vi "BonOMM-SAOMM.vi"() -> ()   [LabVIEW 2019]
uses:
  <vilib>/Utility/miscctls.llb/LVPointTypeDef.ctl
  <vilib>/Utility/miscctls.llb/LVRectTypeDef.ctl
  <vilib>/Analysis/baseanly.llb/Mean (DBL).vi
  SubVIs/Globals.vi
  <vilib>/Utility/config.llb/Read Key (Double).vi
  <vilib>/Utility/config.llb/Read Key (U32).vi
  <vilib>/Utility/config.llb/Read Key (I32).vi
  <vilib>/Utility/config.llb/Read Key (String).vi
  <vilib>/Utility/config.llb/Read Key (Boolean).vi
  SubVIs/Polymorphics/Num2littleEndian(DBL).vi
  SubVIs/Polymorphics/Num2littleEndian(U32).vi
  <vilib>/Instr/_visa.llb/VISA Configure Serial Port (Instr).vi
  SubVIs/Polymorphics/Num2littleEndian(U16).vi
  SubVIs/gfitsio/gfitsio-read-image-subset-sgl-2d.vi
  SubVIs/SAOMM/EXTRACT-DATA-UINT32.vi
  SubVIs/SAOMM/EXTRACT-DATA-UINT16.vi
  SubVIs/SAOMM/EXTRACT-DATA-DBL.vi
  <vilib>/Utility/config.llb/Write Key (Double).vi
  <vilib>/Utility/config.llb/NI_LVConfig.lvlib
  SubVIs/gfitsio/gfitsio.lvlib
  <vilib>/Analysis/NI_AALBase.lvlib
panel:
  in  "VarTab":T1(tab)
  in  "ProcessImage":bool
  out "MaskObjet":u8[][](graph)
  in  "SaveFalconProc":bool
  out "FalconProcData":u8[](array[numeric])
  in  "HexRAZ":bool
  out "Nb_FalconProc_demandé":u32
  in  "GetCommand":string
  out "XROIRef":dbl
  out "YROIRef":dbl
  out "XRefMin":dbl
  out "YRefMin":dbl
  out "XRefMax":dbl
  out "YRefMax":dbl
  out "ROIWidthMin":u16
  out "ROIHeightMin":u16
  out "ROIWidthMax":u16
  out "ROIHeightMax":u16
  out "Nb_Error (PrAMS)":i32
  out "Nb_Error (hex)":i32
  in  "QueryServoLevel":bool
  out "ROISizes":u16[](array[numeric])
  in  "ROIsurface":i32(ring) items=["2.6\" x 2.6\"", "5.2\" x 5.2\"", "7.7\" x 7.7\"", "10.3\" x 10.3\"", "12.9\" x 12.9\"", "20.6\" x 20.6\""]
  out "ROIXMin":u16
  out "ROIYMin":u16
  out "ROIXMax":u16
  out "ROIYMax":u16
  out "PixScale2":dbl=0.323 format="%.4f"
  out "Naxis2":u16=99
  out "Naxis1":u16=142
  out "PixScale1":dbl=0.323 format="%.4f"
  out "Déc étoile guide":dbl=89448.04336960503 caption="DEC" format="%<%H:%M:%S%0u>t"
  out "A.D. étoile guide":dbl=54197.70933641569 caption="RA" format="%<%H:%M:%S%0u>t"
  out "TmpFalcon":u32
  in  "Binning":u16(ring) items=["1 x 1"=1, "2 x 2"=2, "4 x 4"=4, "5 x 5"=5]
  out "FPGA Value":u16(ring) items=["Disabled", "Enabled", "Enabled & Deep Cooling", "Disabled (fan disabled)", "Enabled (fan disabled)", "Enabled & Deep Cooling (fan disabled)"]
  out "InstantFPS":dbl format="%.2f"
  out "HexapodQuery":u32
  out "EMGain":u16
  out "GetOptimalTime":u32
  in  "ImageFPS":dbl=1.0 min=1.0 max=30.0 step=1.0
  out "SetROITime":u32
  out "StartTime":u32
  out "StopTime":u32
  out "SetExpTime":u32
  out "ListenerExec":u32
  out "SetBinningTime":u32
  out "SetFPSTime":u32
  out "ImageWidth":u16
  out "ImageHeight":u16
  out "ROIXOffset":u16
  out "ROIYOffset":u16
  in  "ROIWidth":u16
  in  "ROIHeight":u16
  out "Nb_ACK (PrAMS)":i32
  out "ImageProcessing":u32
  out "FalconQuery":u32
  out "nDumped":i32
  in  "HexapodRefresh":bool
  in  "UpdateROI":bool
  in  "ClearDump":bool
  in  "FalconRefresh":bool
  out "Connexion":bool
  out "Lecture":bool
  out "Écriture":bool
  in  "FalconProcessed":bool
  out "Nb_ACK (hex)":i32
  in  "GetOptimal":bool
  in  "refresh":bool
  out "Nb_FalconProc_reçu":u32
  in  "SendHexOffset":bool caption="SEND Offset"
  out "ImageStat":T2 {"SNR" format="%0.2f"; "mean" format="%0.2f"; "Flux" format="%0.2f"; "Variance" format="%0.2f"; "median" format="%0.2f"}
  out "ImageBuffer":u16[][](graph)
  out "GE_Hex_V":dbl
  out "GE_Hex_U":dbl
  out "GE_Hex_Z":dbl
  out "GE_Hex_Y":dbl
  out "GE_Hex_X":dbl
  out "GE_TCS":bool
  in  "Mode Guidage et Dither":bool=TRUE
  out "MirFOV":dbl=54.5268 caption="Miroir FOV" format="%.2f"
  out "MirVig":dbl=54.5268 caption="Miroir + Vignetting" format="%.2f"
  out "Miroir":dbl=54.5268 format="%.2f"
  in  "ClickJOG":dbl=302.0 min=250.0 max=20000.0
  out "ActiveStages":string[](array[string])
  out "Focusing":bool=TRUE
  out "CurvCorrect":bool=TRUE
  out "CorrectXY":bool=TRUE
  out "CorrectZ":bool=TRUE
  out "MovingZ":bool=TRUE
  out "vitesse jog":dbl=302.0 caption="Vitesse jog" min=250.0 max=20000.0
  out "MovingXY":bool=TRUE
  out "Cible Z":dbl=346504.0
  out "Cible Y":dbl=688453.0
  out "Cible X":dbl=640645.0
  out "NaxisMax":dbl=500000.0 min=-1000000.0 max=1000000.0
  out "Représentation":dbl=54.5268 format="%.2f"
  in  "FoyerAuCentre":dbl=345622.0 min=0.0 max=500000.0 step=10000.0
  in  "a2_focus":dbl=3.3333e-05 format="%.4e"
  in  "a1_focus":dbl=345622.0 min=0.0 max=500000.0 step=10000.0
  out "vitesse focus":dbl=302.0 caption="Vitesse foyer" min=250.0 max=20000.0
  out "RangeTable":dbl=54.5268 format="%.2f"
  out "vitesse lente":dbl=200.0 min=1.0 max=500000.0
  out "vitesse rapide":dbl=30000.0 min=1.0 max=500000.0
  out "accelleration":dbl=200.0 max=1000.0
  in  "a3_focus":dbl=3.3333e-05 format="%.4e"
  in  "k1_focus":dbl=3.3333e-05 format="%.4e"
  in  "k0_focus":dbl=3.3333e-05 format="%.4e"
  out "Position Z":dbl=346504.0
  in  "Calibration X":dbl=624448.0 min=1.0 max=1000000.0
  in  "Calibration Y":dbl=120445.0 max=1000000.0
  in  "Reference X":dbl=669353.0 min=0.0 max=1000000.0
  in  "Reference Y":dbl=53562.0 min=0.0 max=1000000.0
  in  "CentreTel X":dbl=648675.0 min=1.0 max=1000000.0
  in  "CentreTel Y":dbl=37988.0 max=1000000.0
  in  "Rangement X":dbl=1000000.0 min=-1000000.0 max=1000000.0
  in  "Rangement Y":dbl min=-1000000.0 max=1000000.0
  in  "Rangement Z":dbl=500000.0 min=-1000000.0 max=1000000.0
  in  "copy_calib":bool
  in  "copy_ref":bool
  in  "copy_centre":bool
  out "Exceptions":T3={"Command Error"=TRUE, "Slip/Stall"=TRUE, "Overtravel"=TRUE, "Done"=TRUE, "nError"=0, "nSlip"=0, "nOT"=0, "nDone"=0}
  out "Table actif":bool=TRUE
  in  "ApplyCorrection":bool=TRUE
  out "arcsec/pulse":dbl=5.45268e-05 format="%.5e"
  out "LimXPesto":dbl=54.5268 caption="Limit X avec Pesto" format="%.2f"
  in  "GE_TCS_RA":dbl
  in  "GE_TCS_DEC":dbl
  in  "OffsetAcc":dbl caption="Pos" format="%.1f"
  in  "HexYRate":dbl
  in  "HexXRate":dbl
  in  "Offset W":dbl caption="Pos" format="%.6f"
  out "Nominal W":dbl caption="Pos" format="%.4f"
  out "H_Command":dbl[](array[numeric]) format="%.6f"
  out "Cmd X":dbl caption="Pos" format="%.4f"
  out "Cmd Y":dbl caption="Pos" format="%.4f"
  out "Cmd Z":dbl caption="Pos" format="%.4f"
  out "Cmd U":dbl caption="Pos" format="%.4f"
  out "Cmd V":dbl caption="Pos" format="%.4f"
  out "SNRtreshold":dbl caption="ServoSNRTreshold"
  out "QueryTimeStamp":u64
  out "HxMoving":bool caption="Déplacement"
  out "Nominal X":dbl caption="Pos" format="%.4f"
  out "Dump":string
  in  "Signature":u32
  in  "Vitesse [mm/s]":dbl step=10.0 format="%.1f"
  out "Nominal Y":dbl caption="Pos" format="%.4f"
  out "Nominal Z":dbl caption="Pos" format="%.4f"
  out "Nominal U":dbl caption="Pos" format="%.4f"
  out "Nominal V":dbl caption="Pos" format="%.4f"
  out "ActiveLUT":path caption="Look-Up Table active"
  out "H_LUT":dbl[](array[numeric]) format="%.6f"
  out "H_Servo":dbl[](array[numeric]) format="%.6f"
  out "H_Console":dbl[](array[numeric]) format="%.6f"
  out "H_Position":dbl[](array[numeric]) format="%.6f"
  out "H_Offset":dbl[](array[numeric]) format="%.6f"
  out "ConsideredLenght":i32 caption="Considered Data Lenght"
  in  "CorrDelay":u32 caption="Min Delay Between Corrections (ms)"
  in  "LastCorr":u32 caption="Last Correction Occurence"
  in  "CorrTreshold":dbl caption="Correction Treshold"
  in  "RateRA":dbl caption="GuideRateRA"
  in  "BacklashRA":dbl
  in  "RateDEC":dbl caption="GuideRateDEC"
  in  "BacklashDEC":dbl
  in  "Incrément [mm]":dbl step=10.0 format="%.1f"
  out "CorrID":u64 caption="Last Correction ID"
  in  "Offset X":dbl caption="Pos" format="%.6f"
  in  "Offset Y":dbl caption="Pos" format="%.6f"
  in  "Offset Z":dbl caption="Pos" format="%.6f"
  in  "Offset U":dbl caption="Pos" format="%.6f"
  in  "Offset V":dbl caption="Pos" format="%.6f"
  out "Sampling rate":i32 caption="Sampling Rate"
  out "Gain X":dbl caption="Pos" format="%.2f"
  out "Gain Y":dbl caption="Pos" format="%.2f"
  out "Gain Z":dbl caption="Pos" format="%.2f"
  out "Gain U":dbl caption="Pos" format="%.2f"
  out "Gain V":dbl caption="Pos" format="%.2f"
  out "HexW":dbl caption="Pos" format="%.3f"
  out "MessageType":cluster{string[], u32[]}
  out "DiffY":dbl caption="X          Y" format="%.1f"
  out "DiffX":dbl caption="Pos" format="%.1f"
  out "FalconProcTimeStamp":dbl format="%.3f"
  out "LastImageTime":dbl format="%.3f"
  in  "LastImageID":u32
  in  "LastProcID":u64
  out "LastSaveTimeStamp":dbl format="%.3f"
  out "GraphTimeStamp":dbl format="%.3f"
  out "LoggingTimeStamp":dbl format="%.3f"
  out "LastProcSavedID":u64
  out "FieldAstrom":T4 {"CRVAL" format="%.6g"; "CD" format="%_7g"}
  out "TableAstrom":T4 {"CRVAL" format="%.6g"; "CD" format="%_7g"}
  out "ImgAstrom":T4 {"CRVAL" format="%.6g"; "CD" format="%_7g"}
  out "GuiderAstrom":T4 {"CRVAL" format="%.6g"; "CD" format="%_7g"}
  out "tabast_lastmod":timestamp
  out "fldast_lastmod":timestamp
  out "imgast_lastmod":timestamp
  out "RotationEffective":dbl=90.0 caption="Angle du rotateur d'instrument" min=-120.0 max=120.0 step=1.0 format="%.1f"
  in  "Ajustement fin de rotation":dbl=-0.27
  out "HA":dbl
  out "DEC":dbl format="%.10g"
  in  "BoutonTest":bool
  in  "DC_button":bool
  out "DC String":string="   3.999928\r  19.539602\r   9.999081\r2008.731741\r   2.122384\r  23.539530\r   4.058605\r2008.731741\r3395.000000\r 133.394864\r  90.000000\r"
  in  "Numero_DC":string caption="Instrument Actuel"
  in  "Dec_DC":string="9:59:57" caption="Déclinaison du prochain objet"
  in  "AD_DC":string="19:30:53" caption="Ascension Droite du prochain objet"
  in  "Nom_DC":string caption="Instrument Actuel"
  out "StateGuidageDither":bool
  out "Guidage en cour":bool=TRUE
  in  "QuitInitialization":bool
  out "TCSMute":bool
  out "GuidingCancel":bool
  out "Offset en cours":bool
  out "SplitterMoving":bool
  out "ReconnectionMute":bool
  out "SaveNextImage":bool
  out "TableMute":bool
  out "QueryingHexapod":bool=TRUE
  out "Quit_Origine":bool
  out "Hexapod-Error":bool=TRUE
  out "PrAMS-Error":bool=TRUE
  out "HexaSpam":bool=TRUE
  out "Hexapod-ACK":i32
  out "HexaCons actif":bool=TRUE
  out "QueryingPraMS":bool=TRUE
  out "PrAMS-ACK":i32
  out "PrAMS actif":bool=TRUE
  out "Origine en cours...":bool
  out "SubIMG4DSS?":bool=TRUE
  out "Centrage_ready":bool=TRUE
  in  "DS9_ready":bool
  out "Offset DEC clic-sim":bool
  out "Offset RA clic-sim":bool
  out "NO RA clic-sim":bool
  out "NeedOrigin":bool
  in  "CursorLock":bool
  out "FirstBest":bool
  out "cRIO Port":u16
  out "Librairie complète":string[][](table)=[["1", "WR1", "00:43:28", "64:45:35", "2000.0", "1.153488"], ["2", "WR2", "01:05:23", "60:25:18", "2000.0", "1.142985"], ["3", "WR3", "02:54:30", "-10:00:17", "2006.2", "2.742240"], ["4", "WR4", "02:00:00", "10:00:00", "2000.0", "1.613543"], ["5", "WR5", "02:52:11", "56:56:07", "2000.0", "1.148727"], ["6", "WR6", "06:54:13", "-23:55:42", "2000.0", "7.346970"], ["7", "WR7", "07:18:29", "-13:13:01", "2000.0", "3.540250"], ["8", "WR7a", "07:20:22", "-23:43:57", "2000.0", "7.387993"], ["9", "WR8", "07:44:58", "-31:54:29", "2000.0", "29.253050"]]
  out "Q String":string="   3.999928\r  19.539602\r   9.999081\r2008.731741\r   2.122384\r  23.539530\r   4.058605\r2008.731741\r3395.000000\r 133.394864\r  90.000000\r"
  out "TabQstr":string="    688453,    640645,    346504,         0,K,K,R\r"
  out "Éléments cochés":bool[](array[boolean])
  in  "SaveExcpt":bool
  in  "Tableau des exceptions":string[](array[string])=["TERMINAL"]
  out "cRIO_commID":refnum<k5>
  in  "modify-librairy":bool
  out "cRIO address":string="132.204.61.43"
  out "Exception":string[](array[string])=["TERMINAL"]
  out "CtrlName":string[](array[string])=["Origine", "Quit", "Vitesse de jog", "v rapide", "v lent", "RangeTablesXY", "Focus Low Speed", "Mode", "Temps\nexp.", "GoCam", "stoptable", "Focus High Speed", "NumberofImg", "Binning", "XÉtoile", "YÉtoile", "Acceleration Time", "TempRefresh", "GuidePixScale", "Initialise\nTCS", "Synctel", "ModifRotation", "StopTel", "N.O. A.D.", "ModifFoyer", "Calibration", "Z Min", "Z Max", "Autoscale", "Range\nTélescope", "Zénith", "RangeTable", "ModCoor", "StopCam", "sonde?", "Écran", "OffrotChamp", "Éléments du menu Autres commandes", "Éléments du menu affichage", "k planfocal", "CenCurs", "Mode TimeOut", "ModifDome", "SyncDome-Tél", "Coupole-Tél", "VTel", "CentreTel Y", "CentreTel X", "PauseCAM", "Zfine+", "Zfine-", "Set angle", "AngOK", "PAS", "ANG+", "ANG-", "Centrage", "go Est", "go Nord", "go Ouest", "go Sud", "Offrot Calib", "Mise à jour", "FoyerCentre", "Foyer+", "Foyer-", "Offset OK", "Déplacer sonde ?", "Offset Déc.", "Offset A.D.", "Historique des observations", "Table Baud rate", "TCS C Baud rate", "Calib Baud rate", "Excmd Baud rate", "TCS R Baud rate", "Calib VRN", "Excmdl VRN", "Table VRN", "TCS R VRN", "TCS C VRN", "Rapport focal", "Flat", "Néon", "Arc", "Tableau des filtres", "Charger l'objet sélectionné", "Pos Y (centre)", "Pos X (centre)", "Pos X (calibration)", "Pos Y (calibration)", "Pos Y (rangement)", "Pos X (rangement)", "Pos Z (rangement)", "vitesse lente", "vitesse rapide", "accelleration", "CamCooler", "TemperatureSetpoint", "Rafraîchir Image", "z-spd-slide", "Rayon de sécurité ...", "load-histo(L)", "Alarme Humidité", "Alarme Température", "Alarme D humidité", "Alarme vent", "Alarme D température", "modif-alarm-param", "Alarme point de rosée", "save-parametres", "BIN_IMG", "Use-focus-comp?", "Rot(CAM)", "ScopeSim._Telescope", "MaxIm.ICCDCamera", "MC-BonOMM VRN", "ST_SPD", "Load-library", "modify-librairy", "DS-CID", "string temporaire", "Ajust z to tel", "Époque", "N.O. Déc.", "tab panel", "GO", "ChoixFiltre", "change_filtre_liste", "q-raf", "cancel-raf", "reconnect", "Périphérique", "ST+", "ST-", "SET ZERO", "ST_RAZ", "Alacible", "Centre", "X.agg", "Y.agg", "centrer_curseur_table", "error out (property node)", "error out (RefNum open)", "SaveExcpt", "Tableau des exceptions", "Use_tuning?", "Recalculer", "Sécurité Exclusion", "Save time", "Last save"]
  out "menu ref":refnum<k9>
  out "TCS C actif":bool
  out "TCS actif":bool
  out "Downloading ...":bool
  out "DSS_ready":bool
  out "USNO_ready":bool
  in  "Recalculer":bool
  out "DST?":bool
  out "CursorGrab":bool
  out "imageDSS":bool
  out "Déplacement usager":bool
  out "Bypass Auto-focus":bool
  out "From library":bool
  out "Annulation en cours":bool
  out "Bypass Tech":bool
  out "Annulation du foyer":bool
  out "Mode Est":bool
  out "FIFO actif":bool
  out "AutoConnect?":bool
  in  "Sync_Ready":bool=TRUE
  in  "Setting":bool
  out "Origin":T5
  out "Front Panel Window:Panel Bounds":T6
  out "Front Panel Window:Minimum Size":T5
  in  "Coupole-Tél":bool
  in  "ForceSaveToFile":bool
  out "SkipChoixInstr":bool
  in  "LVDT-RA-Data":dbl[](array[numeric])
  out "Status lamp":bool[](array[boolean])
  out "section names":string[](array[string])
  in  "ANG-":bool
  in  "ANG+":bool
  in  "PAS":dbl format="%.2f"
  in  "AngOK":bool
  in  "Set angle":dbl format="%.2f"
  in  "string temporaire":string="Bleu\nVisible\nrien\nblank\nblank\nblank\n"
  in  "Tableau des filtres":string[](array[string])=["VIDE", "ESPIOMM ROUGE", "ESPIOMM BLEU", "R SDSS", "R STANDARD", ""]
  out "Ath_coef":dbl=3450.0 caption="Coefficient d'athermalisation" format="%.2f"
  out "Foyer Nominal":dbl=3450.0 format="%.2f"
  out "tmp.str":dbl=3450.0 caption="Temp. Serrurier" format="%.2f"
  out "last_foc_chg":ext=650514.5633458178 format="%.2f"
  out "CheckFocus":bool
  out "Foyer Avant":dbl=3450.0 format="%.2f"
  in  "LVDT-time":dbl=0.05
  in  "LVDT-zero":dbl
  out "LVDT-RA":refnum<k21>
  in  "ZeroRAZ":bool
  in  "DECRAZ":bool
  in  "Clear":bool
  in  "LVDT-scale":dbl
  out "Graph Data":dbl[](array[numeric])
  out "Graph-SNR":cluster{dbl[], dbl[]}[](graph)=[{[3293923535.3589997, 3293923538.453, 3293923543.125, 3293923547.3589997, 3293923551.6089997, 3293923555.562, 3293923592.9059997, 3293923596.875, 3293923600.812, 3293923604.546, 3293923608.9839997, 3293923612.968, 3293923616.812, 3293923620.6559997, 3293923624.25, 3293923628.093, 3293923631.468, 3293923635.718, 3293923639.671, 3293923643.9059997, 3293923648.093, 3293923651.796, 3293923655.64, 3293923659.312, 3293923670.14, 3293923673.828, 3293923677.75, 3293923688.062, 3293923722.5309997, 3293923726.64, 3293923730.671, 3293923734.843, 3293923739.015, 3293923743.437, 3293923747.437], [0.19257166981697083, 0.19257166981697083, 0.42606911063194275, 0.5051353573799133, 0.24072398245334625, -0.04916790872812271, -0.10410226881504059, -0.10410226881504059, 0.34198060631752014, -0.09570426493883133, 0.19647449254989624, 0.3240731954574585, -0.04466410353779793, -0.24122145771980286, -0.010196941904723644, -0.010196941904723644, 0.0218539796769619, 0.0218539796769619, 0.16859716176986694, 0.37170615792274475, 0.37170615792274475, 0.26590290665626526, 0.026526281610131264, 0.2402668595314026, -0.03137940168380737, -0.024852409958839417, -0.08229449391365051, -0.2815259099006653, -0.8884221911430359, -0.4433065354824066, -1.0303088426589966, -0.24918021261692047, -0.3698801100254059, 0.029610345140099525, 0.7200243244171143]}, {[3293923535.3589997, 3293923538.453, 3293923543.125, 3293923547.3589997, 3293923551.6089997, 3293923555.562, 3293923592.9059997, 3293923596.875, 3293923600.812, 3293923604.546, 3293923608.9839997, 3293923612.968, 3293923616.812, 3293923620.6559997, 3293923624.25, 3293923628.093, 3293923631.468, 3293923635.718, 3293923639.671, 3293923643.9059997, 3293923648.093, 3293923651.796, 3293923655.64, 3293923659.312, 3293923670.14, 3293923673.828, 3293923677.75, 3293923688.062, 3293923722.5309997, 3293923726.64, 3293923730.671, 3293923734.843, 3293923739.015, 3293923743.437, 3293923747.437], [0.02463431842625141, 0.02463431842625141, 0.33257317543029785, -0.26877567172050476, -0.21053607761859894, -0.3878229558467865, -0.627870500087738, -0.627870500087738, -0.35187196731567383, 0.61182701587677, 0.414733350276947, 0.06820612400770187, 0.033184804022312164, 0.28442147374153137, 0.3806324601173401, 0.3806324601173401, -0.5958633422851562, -0.5958633422851562, -0.3973797857761383, 0.1421676129102707, 0.1421676129102707, 0.390238881111145, 0.4161102771759033, 0.6681324243545532, 0.08439777046442032, 0.12898856401443481, 0.07825367152690887, -0.09022828936576843, -0.0057562836445868015, -0.2819269895553589, -0.21260638535022736, 0.050426241010427475, -0.3064248561859131, 0.3770900368690491, 0.3633768482208252]}]
  out "Cumulatif":cluster{dbl[], dbl[]}[](graph)
  out "HexYData":cluster{dbl[], dbl[]}[](array[cluster])
  out "HexXData":cluster{dbl[], dbl[]}[](array[cluster])
  out "SNRData":cluster{dbl[], dbl[]}[](array[cluster])
  out "FluxData":cluster{dbl[], dbl[]}[](array[cluster])
  out "CentroidsData":cluster{dbl[], dbl[]}[](array[cluster])
  out "CumulativeError":cluster{dbl[], dbl[]}[](array[cluster])
  out "SetVOffset":bool
  out "SetUOffset":bool
  in  "DefaultUAxisOffset":dbl=0.27
  in  "DefaultVAxisOffset":dbl=0.27
  out "RA-USNO-sec 3":dbl=70342.56719999999 caption="RA-Champ" format="%<%H:%M:%S%1u>t"
  out "RA-USNO-sec 2":dbl=70342.56719999999 caption="RA-Champ" format="%<%H:%M:%S%1u>t"
  out "DEC-Champ-sec":dbl=70342.56719999999 caption="RA-Champ" format="%<%H:%M:%S>t"
  out "RA-Champ-sec":dbl=70342.56719999999 caption="RA-Champ" format="%<%H:%M:%S%1u>t"
  out "Target Data":string[][](array[string])
  out "dflt-EQX":dbl=2008.731741 caption="Default-EQUINOX" format="%.8f"
  out "STATEX":bool[](array[boolean])
  out "STATLH":bool[](array[boolean])=[FALSE, TRUE, FALSE, FALSE, FALSE, FALSE, FALSE, FALSE, FALSE, FALSE, FALSE, FALSE, FALSE, FALSE, FALSE, FALSE, FALSE, FALSE, FALSE, FALSE, FALSE, FALSE, FALSE, FALSE, FALSE, FALSE, FALSE, FALSE, FALSE, FALSE, FALSE, FALSE]
  out "STATH":bool[](array[boolean])=[FALSE, FALSE, TRUE, FALSE, FALSE, TRUE, TRUE, TRUE, FALSE, FALSE, FALSE, FALSE, FALSE, FALSE, FALSE, FALSE, FALSE, FALSE, FALSE, FALSE, FALSE, FALSE, FALSE, FALSE, FALSE, FALSE, FALSE, FALSE, FALSE, FALSE, FALSE, FALSE]
  out "STATL":bool[](array[boolean])=[TRUE, FALSE, FALSE, FALSE, FALSE, FALSE, FALSE, FALSE, FALSE, FALSE, FALSE, FALSE, FALSE, FALSE, FALSE, FALSE, FALSE, FALSE, FALSE, FALSE, FALSE, FALSE, FALSE, FALSE, FALSE, FALSE, FALSE, FALSE, FALSE, FALSE, FALSE, FALSE]
  out "USNO_data":string[][](array[string])
  out "DEC-USNO":dbl=35996.6916 caption="DEC-USNO  [°]" format="%.6f"
  out "RA-USNO":dbl=70342.56719999999 caption="RA-USNO  [°]" format="%.6f"
  out "RA-Champ":dbl=70342.56719999999 format="%.6f"
  out "DEC-Champ":dbl=70342.56719999999 format="%.6f"
  out "Img DEC":dbl=35996.6916 caption="ImgDEC  [°]" format="%.6f"
  out "Img RA":dbl=70342.56719999999 caption="ImgRA  [°]" format="%.6f"
  out "ImgData":sgl[][](array[numeric])
  out "Path2Image":path
  out "DEC-USNO-sec":dbl=70342.56719999999 caption="RA-Champ" format="%<%H:%M:%S>t"
  out "RA-USNO-sec":dbl=70342.56719999999 caption="RA-Champ" format="%<%H:%M:%S%1u>t"
  out "DEC-DSS-sec":dbl=70342.56719999999 caption="RA-Champ" format="%<%H:%M:%S>t"
  out "RA-DSS-sec":dbl=70342.56719999999 caption="RA-Champ" format="%<%H:%M:%S%1u>t"
  out "AnnéeRL":dbl=2008.731741 format="%.8f"
  out "RAtmp":dbl=70342.5708 format="%<%H:%M:%S%2u>t"
  out "Dectmp":dbl=35996.688 format="%<%H:%M:%S%2u>t"
  in  "BestCount":i32
  out "HexapodeTempError":errorcluster
  out "PrAMS Error":errorcluster
  out "LVDT Error":errorcluster
  out "TCS #26 (sort)":u32
  out "TimeBetweenExec":u32
  out "DSS Error":errorcluster
  out "Meteo Error":errorcluster
  out "File I/O Error":errorcluster
  out "Config Error":errorcluster
  out "TCS Error":errorcluster
  out "Table Error":errorcluster
  out "Critical Error":errorcluster
  out "ActiveX Error":errorcluster
  out "Guider Error":errorcluster
  out "Excom Error":errorcluster
  in  "FIFO d'erreur":T7(array[cluster])
  out "IndicSetErrInd":bool
  out "CtrlGetErrInd":bool
  out "CtrlSetError":errorcluster[](array[cluster])
  out "IndicSetError":errorcluster[](array[cluster])
  out "wget error":errorcluster
  out "TCP/IP Error":errorcluster
  out "Serial Error":errorcluster
  out "Menu Error":errorcluster
  out "VI Reference Error":errorcluster
  out "Starry Night Error":errorcluster
  out "TotalExecTime":u32
  out "CommCheck":u32
  out "Wait4Flag":u32
  out "TCS #26":u32
  out "TCS #25":u32
  out "Table Q":u32
  out "CursorSet":u32
  out "fits Error":errorcluster
  out "AS_I_Pillier":bool
  in  "AS_B_Pillier":bool
  in  "MainTab":T8(tab)
  in  "BrasPesto":bool=TRUE caption="Bras de pesto\n déployé"
  out "LowSNR":bool
  out "GuideWest":bool
  out "GuideSouth":bool
  out "GuideEast":bool
  out "GuideNorth":bool
  out "EcartV":dbl caption="Écart V" format="%.4f"
  out "EcartU":dbl caption="Écart U" format="%.4f"
  out "EcartZ":dbl caption="Écart Z" format="%.4f"
  out "EcartY":dbl caption="Écart Y" format="%.4f"
  out "EcartX":dbl caption="Écart X" format="%.4f"
  out "Alarme PRAMS":bool
  out "Tracking":bool caption="En déplacement"
  out "FOV":dbl caption="Champ de vue instrumental" format="%.1f"
  out "Instrument Actuel":string
  in  "Synctel":bool caption="Synchronisation des coordonnées"
  in  "Range":bool
  in  "Zénith":bool
  in  "Écran":bool
  out "Focus slew":bool caption="Foyer en déplacement"
  out "Slew enabled":bool caption="Prêt à pointer"
  out "Slewing":bool caption="En déplacement"
  in  "StopTel":bool caption="Stop - Télescope"
  in  "GO":bool caption="GO - Telescope"
  out "LST":dbl=84742.30799999999 caption="Temps Sidéral" format="%<%H:%M:%S%0u>t"
  out "UTC":dbl=14610.978 caption="Temps Universel" format="%<%H:%M:%S%0u>t"
  in  "ModifDome":bool caption="Initialisation du dôme"
  out "Coupole":dbl=133.394864 min=0.0 max=359.0 step=1.0
  in  "ModifFoyer":bool caption="Foyer du télescope"
  in  "ModifRotation":bool caption="Rotation de la bonnette"
  out "Foyer":dbl=3395.0 caption="Relacher pour \nmodifier TCS"
  in  "ModCoor":bool caption="Charger les coordonnées"
  out "NO HA":dbl=14399.740800000001 caption="Angle Horaire du prochain objet" format="%<%H:%M:%S%1u>t"
  out "NO AM":dbl=2.122384 caption="Masse d'air du prochain objet" format="%.2f"
  in  "NO epoch":dbl=2008.72901 caption="Équinoxe du prochain objet" format="%.2f"
  in  "N.O. Déc.":string="9:59:57" caption="Déclinaison du prochain objet"
  in  "N.O. A.D.":string="19:30:53" caption="Ascension Droite du prochain objet"
  out "Epoch Tel":dbl=2008.731741 caption="Époque" format="%.2f"
  out "Angle Hor.":dbl=14399.740800000001 caption="Angle Horaire du Télescope" format="%<%H:%M:%S%1u>t"
  out "DEC Tel":dbl=35996.6916 caption="Déclinaison du Télescope" format="%<%H:%M:%S%0u>t"
  out "RA Tel":dbl=70342.56719999999 caption="Ascension Droite du Télescope" format="%<%H:%M:%S%1u>t"
  out "Air Mass":dbl=2.122384 caption="Masse d'air du télescope" format="%.2f"
  in  "SaveCoords":bool caption="Enregistrer la position actuelle"
  out "Foyer à 0°":i32
  out "Dec Cible":dbl=34150.93098198265 format="%<%H:%M:%S%0u>t"
  out "RA Cible":dbl=70407.26510530974 caption="RA de la Cible" format="%<%H:%M:%S%1u>t"
  out "Dec Sonde":dbl=34150.89703708518 caption="DEC de la sonde" format="%<%H:%M:%S%0u>t"
  out "RA Sonde":dbl=70407.2665759738 caption="RA de la sonde" format="%<%H:%M:%S%1u>t"
  in  "centrer_curseur_table":bool caption="Placer la cible sur la position actuelle"
  in  "Ajust z to tel":bool caption="Ajustement automatique du foyer"
  in  "FoyerTable":dbl=346504.0 caption="Foyer de guidage" min=0.0 max=1000000.0 step=1.0 format="%#.0f"
  in  "centrer_curseur":bool caption="Centrer le curseur"
  in  "go Sud":bool caption="Ajustement Sud"
  in  "go Est":bool caption="Ajustement Est"
  in  "go Nord":bool caption="Ajustement Nord"
  in  "go Ouest":bool caption="Ajustement Ouest"
  in  "enfoncé":bool
  in  "Foyer+":bool caption="Foyer +"
  in  "Foyer-":bool caption="Foyer -"
  out "act_cible":bool caption="Cible Active"
  out "act_sonde":bool caption="Sonde Active"
  out "OffRA_dir":string caption="Direction du offset (A.D.)"
  in  "Offset OK":bool
  in  "Offset DEC":dbl caption="DEC" format="%.1f"
  in  "Offset RA":dbl=-30.0 caption="A.D." format="%.1f"
  out "OffDEC_dir":string caption="Direction du offset (Dec.)"
  in  "GetDSS":bool caption="Champ DSS"
  in  "best_target":bool caption="Meilleure Cible"
  in  "DS9":bool caption="Repérage (finding chart)"
  out "subimg":sgl[][](graph) caption="Région d'intérêt (ROI)"
  out "Cen-Cib-TOT":string caption="Distance au centre de la cible (total)"
  in  "Cen-Cib-DEC":string caption="Distance au centre de la cible (DEC)"
  in  "Cen-Cib-RA":string caption="Distance au centre de la cible (RA)"
  out "Cen-Snd-TOT":string caption="Distance au centre de la sonde (total)"
  out "Cen-Snd-DEC":string caption="Distance au centre de la sonde (DEC)"
  out "Cen-Snd-RA":string caption="Distance au centre de la sonde (RA)"
  out "TableXYPos":cluster{dbl[], dbl[]}[](graph) caption="Représentation du champ"
  in  "Centrage":bool caption="Routine de Centrage"
  in  "Alacible":bool caption="À la cible"
  in  "Origine":bool
  in  "Calibration":bool
  in  "RangeTable":bool caption="Rangement"
  in  "stoptable":bool caption="Arrêt d'urgence des tables"
  out "ImageDSSLed":bool
  out "BestTargetLed":bool
  out "DS9-Led":bool
  out "CentrageLed":bool
  in  "CameraSelector":T9(tab)
  in  "Milieu":bool caption="Prendre le centroïde comme référence"
  out "ErrX":string caption="Résidu Y"
  out "SNR":dbl=1.0 min=0.0 max=60.0 step=1.0 format="%.1f"
  in  "AutoCentroid":bool caption="Prendre le centroïde comme référence"
  out "Picture":picture
  out "ImgArray":u32[][](graph) caption="Image de la Falcon"
  in  "exptime":dbl=1.0 caption="Temps d'exposition" min=0.0 max=60.0 step=1.0 format="%.3f"
  in  "GoCam":bool caption="Démarrer l'exposition"
  in  "StopCam":bool caption="Arrêter l'exposition"
  out "Integrating":bool caption="Integration"
  in  "Mode":u16(ring)=2 items=["Opération Fixe (Guidage traditionnel)", "Asservissement Passif (LUT + Guidage)", "Asservissement Actif (LUT + Servo + Guidage)", "Collimation", "Guidage externe", ""]
  in  "StopServo":bool caption="Stop"
  in  "StartServo":bool caption="Go"
  out "Servo":bool
  in  "XReference":dbl caption="Pixel de Référence X" format="%.1f"
  in  "YReference":dbl caption="Pixel de Référence Y" format="%.1f"
  out "XCentroid":dbl caption="Pos" format="%.1f"
  out "YCentroid":dbl caption="Centroïd X" format="%.1f"
  out "ErrY":string caption="Résidu X"
  in  "Corr%":dbl=75.0 caption="Aggressivité" min=5.0 max=125.0 step=5.0 format="%.0f %"
  out "LUT V":dbl caption="Pos" format="%.4f"
  out "LUT U":dbl caption="Pos" format="%.4f"
  out "LUT Z":dbl caption="Pos" format="%.4f"
  out "LUT Y":dbl caption="Pos" format="%.4f"
  out "LUT X":dbl caption="Pos" format="%.4f"
  out "LUT W":dbl caption="Pos" format="%.4f"
  out "Hex-YGraph":cluster{dbl[], dbl[]}[](graph) caption="Graphique de la position de l'Hexapode X"
  out "Hex-XGraph":cluster{dbl[], dbl[]}[](graph) caption="Graphique de la position de l'Hexapode Y"
  in  "SpliterSelector":u16(ring) items=["Initialisation", "Retirer la lame séparatrice du faisceau", "Mettre la lame séparatrice dans le faisceau"]
  out "SpliterIndic":bool
  out "Flux Min":dbl=912473.0
  out "Flux Max":dbl=912473.0
  out "Flux inst.":dbl=341382.0
  out "Histogramme de la ROI":T10(graph)
  out "PSF Graph":cluster{"PSF X":dbl[], "PSF Y":dbl[]}[](graph) caption="Graphique de la PSF"
  out "Seeing":dbl caption="Scintillation" format="%.2g"
  in  "HautDroit":T11(tab)
  out "MC_connect":bool=TRUE
  in  "Périphérique":u16(ring) caption="Sélection du périphérique" items=["Roue à Filtres (BonOMM)", "Roue à Filtres (PANO-II)", "Foyer ST-133", "Lampes d'étalonnage", "Options des périphériques"]
  out "filtre_nom":string="ESPIOMM ROUGE"
  out "F#":i32=2 caption="Filtre"
  in  "cancel-raf":bool
  in  "q-raf":bool
  in  "change_filtre_liste":bool
  in  "ChoixFiltre":T12
  in  "reconnect":bool
  in  "Arc":bool
  in  "Néon":bool
  in  "Flat":bool
  in  "ST_SPD":dbl(slide)=34.285714285714285 caption="vitesse (%)" min=1.0 max=100.0 scale=0.0..100.0
  in  "SET ZERO":bool
  in  "ST_RAZ":bool
  in  "ST+":bool
  in  "ST-":bool
  in  "Obslib":string[][](table)=[["7:11:00", "24:49:54", "2008.73", "04:12", "", "", "", "", ""], ["7:10:47", "24:50:15", "2008.73", "04:05", "", "", "", "", ""], ["2:37:38", "61:38:54", "2008.73", "22:53", "2:36:49", "60:58:56", "279", "162", "guidage lancé à \"heure\""], ["21:22:31", "45:59:16", "2008.73", "22:33", "", "", "", "", ""], ["21:20:55", "45:53:43", "2008.73", "22:32", "", "", "", "", ""], ["21:20:42", "45:51:12", "2008.73", "21:55", "", "", "", "", ""], ["20:56:28", "31:29:45", "2008.73", "21:40", "20:54:55", "31:23:11", "514", "15", "guidage lancé à \"heure\""]] caption="Historique des observations"
  in  "Load_obj":bool caption="Charger l'objet sélectionné"
  out "Cx":bool=TRUE caption="cRIO_comm"
  out "indic-T-struct":dbl=8.517964858102035 caption="Miroir" format="%.1f"
  out "indic-Tm":dbl=8.517964858102035 caption="Miroir" format="%.1f"
  out "indic-H-out":dbl=78.14770167340113 format="%.1f"
  out "indic-H-in":dbl=63.74411594905159 format="%.1f"
  out "indic-T-out":dbl=5.6293850395316785 format="%.1f"
  out "indic-T-in":dbl=8.455195486699632 format="%.1f"
  out "Hexapode Temperatures":T13
  out "Hexapod Alarms":bool[](array[boolean])
  out "LVDT-DEC-inst":dbl format="%.3f"
  in  "LVDT-Set-ZERO":bool
  out "LVDT-RA-closeup":cluster{dbl, dbl, dbl[]}(graph)
  out "LVDT-RA-coarse":cluster{dbl, dbl, dbl[]}(graph)
  in  "LVDT-Save-Data":bool
  out "LVDT-RA-inst":dbl format="%.3f"
  out "Guiderreur":cluster{dbl[], dbl[]}[](graph)=[{[-0.950748243115165, -0.7916270440275018, -0.6325058449398387, -0.4733846458521756, -0.3142634467645125, -0.15514224767684937, 0.0039789514108137655, 0.1631001504984769, 0.32222134958614, 0.48134254867380316, 0.6404637477614663], [-3.0, -5.0, -5.0, -4.0, -1.0, -1.0, 5.0, 1.0, 0.0, -3.0, -4.0]}, {[0.0, -3.75, 0.0, -1.25, -3.75, 3.75, 0.0, -3.75, 5.0, -5.0, -2.5], [-0.568961276249452, -0.45114282857288013, -0.3333243808963082, -0.21550593321973627, -0.09768748554316434, 0.020130962133407593, 0.13794940980997952, 0.25576785748655145, 0.3735863051631234, 0.4914047528396953, 0.6092232005162672]}, {[0.19257166981697083, 0.19257166981697083, 0.42606911063194275, 0.5051353573799133, 0.24072398245334625, -0.04916790872812271, -0.10410226881504059, -0.10410226881504059, 0.34198060631752014, -0.09570426493883133, 0.19647449254989624, 0.3240731954574585, -0.04466410353779793, -0.24122145771980286, -0.010196941904723644, -0.010196941904723644, 0.0218539796769619, 0.0218539796769619, 0.16859716176986694, 0.37170615792274475, 0.37170615792274475, 0.26590290665626526, 0.026526281610131264, 0.2402668595314026, -0.03137940168380737, -0.024852409958839417, -0.08229449391365051, -0.2815259099006653, -0.8884221911430359, -0.4433065354824066, -1.0303088426589966, -0.24918021261692047, -0.3698801100254059, 0.029610345140099525, 0.7200243244171143], [0.02463431842625141, 0.02463431842625141, 0.33257317543029785, -0.26877567172050476, -0.21053607761859894, -0.3878229558467865, -0.627870500087738, -0.627870500087738, -0.35187196731567383, 0.61182701587677, 0.414733350276947, 0.06820612400770187, 0.033184804022312164, 0.28442147374153137, 0.3806324601173401, 0.3806324601173401, -0.5958633422851562, -0.5958633422851562, -0.3973797857761383, 0.1421676129102707, 0.1421676129102707, 0.390238881111145, 0.4161102771759033, 0.6681324243545532, 0.08439777046442032, 0.12898856401443481, 0.07825367152690887, -0.09022828936576843, -0.0057562836445868015, -0.2819269895553589, -0.21260638535022736, 0.050426241010427475, -0.3064248561859131, 0.3770900368690491, 0.3633768482208252]}] caption="Histogramme de guidage"
  out "Graph-Centroids":cluster{"TimeArray":dbl[], dbl[]}[](graph)=[{"TimeArray"=[3293923535.3589997, 3293923538.453, 3293923543.125, 3293923547.3589997, 3293923551.6089997, 3293923555.562, 3293923592.9059997, 3293923596.875, 3293923600.812, 3293923604.546, 3293923608.9839997, 3293923612.968, 3293923616.812, 3293923620.6559997, 3293923624.25, 3293923628.093, 3293923631.468, 3293923635.718, 3293923639.671, 3293923643.9059997, 3293923648.093, 3293923651.796, 3293923655.64, 3293923659.312, 3293923670.14, 3293923673.828, 3293923677.75, 3293923688.062, 3293923722.5309997, 3293923726.64, 3293923730.671, 3293923734.843, 3293923739.015, 3293923743.437, 3293923747.437], [0.19257166981697083, 0.19257166981697083, 0.42606911063194275, 0.5051353573799133, 0.24072398245334625, -0.04916790872812271, -0.10410226881504059, -0.10410226881504059, 0.34198060631752014, -0.09570426493883133, 0.19647449254989624, 0.3240731954574585, -0.04466410353779793, -0.24122145771980286, -0.010196941904723644, -0.010196941904723644, 0.0218539796769619, 0.0218539796769619, 0.16859716176986694, 0.37170615792274475, 0.37170615792274475, 0.26590290665626526, 0.026526281610131264, 0.2402668595314026, -0.03137940168380737, -0.024852409958839417, -0.08229449391365051, -0.2815259099006653, -0.8884221911430359, -0.4433065354824066, -1.0303088426589966, -0.24918021261692047, -0.3698801100254059, 0.029610345140099525, 0.7200243244171143]}, {"TimeArray"=[3293923535.3589997, 3293923538.453, 3293923543.125, 3293923547.3589997, 3293923551.6089997, 3293923555.562, 3293923592.9059997, 3293923596.875, 3293923600.812, 3293923604.546, 3293923608.9839997, 3293923612.968, 3293923616.812, 3293923620.6559997, 3293923624.25, 3293923628.093, 3293923631.468, 3293923635.718, 3293923639.671, 3293923643.9059997, 3293923648.093, 3293923651.796, 3293923655.64, 3293923659.312, 3293923670.14, 3293923673.828, 3293923677.75, 3293923688.062, 3293923722.5309997, 3293923726.64, 3293923730.671, 3293923734.843, 3293923739.015, 3293923743.437, 3293923747.437], [0.02463431842625141, 0.02463431842625141, 0.33257317543029785, -0.26877567172050476, -0.21053607761859894, -0.3878229558467865, -0.627870500087738, -0.627870500087738, -0.35187196731567383, 0.61182701587677, 0.414733350276947, 0.06820612400770187, 0.033184804022312164, 0.28442147374153137, 0.3806324601173401, 0.3806324601173401, -0.5958633422851562, -0.5958633422851562, -0.3973797857761383, 0.1421676129102707, 0.1421676129102707, 0.390238881111145, 0.4161102771759033, 0.6681324243545532, 0.08439777046442032, 0.12898856401443481, 0.07825367152690887, -0.09022828936576843, -0.0057562836445868015, -0.2819269895553589, -0.21260638535022736, 0.050426241010427475, -0.3064248561859131, 0.3770900368690491, 0.3633768482208252]}] caption="Graphique des Centroïdes"
  out "Graph-Flux":cluster{"TimeArray":dbl[], dbl[]}[](graph)=[{"TimeArray"=[3293923535.3589997, 3293923538.453, 3293923543.125, 3293923547.3589997, 3293923551.6089997, 3293923555.562, 3293923592.9059997, 3293923596.875, 3293923600.812, 3293923604.546, 3293923608.9839997, 3293923612.968, 3293923616.812, 3293923620.6559997, 3293923624.25, 3293923628.093, 3293923631.468, 3293923635.718, 3293923639.671, 3293923643.9059997, 3293923648.093, 3293923651.796, 3293923655.64, 3293923659.312, 3293923670.14, 3293923673.828, 3293923677.75, 3293923688.062, 3293923722.5309997, 3293923726.64, 3293923730.671, 3293923734.843, 3293923739.015, 3293923743.437, 3293923747.437], [0.19257166981697083, 0.19257166981697083, 0.42606911063194275, 0.5051353573799133, 0.24072398245334625, -0.04916790872812271, -0.10410226881504059, -0.10410226881504059, 0.34198060631752014, -0.09570426493883133, 0.19647449254989624, 0.3240731954574585, -0.04466410353779793, -0.24122145771980286, -0.010196941904723644, -0.010196941904723644, 0.0218539796769619, 0.0218539796769619, 0.16859716176986694, 0.37170615792274475, 0.37170615792274475, 0.26590290665626526, 0.026526281610131264, 0.2402668595314026, -0.03137940168380737, -0.024852409958839417, -0.08229449391365051, -0.2815259099006653, -0.8884221911430359, -0.4433065354824066, -1.0303088426589966, -0.24918021261692047, -0.3698801100254059, 0.029610345140099525, 0.7200243244171143]}, {"TimeArray"=[3293923535.3589997, 3293923538.453, 3293923543.125, 3293923547.3589997, 3293923551.6089997, 3293923555.562, 3293923592.9059997, 3293923596.875, 3293923600.812, 3293923604.546, 3293923608.9839997, 3293923612.968, 3293923616.812, 3293923620.6559997, 3293923624.25, 3293923628.093, 3293923631.468, 3293923635.718, 3293923639.671, 3293923643.9059997, 3293923648.093, 3293923651.796, 3293923655.64, 3293923659.312, 3293923670.14, 3293923673.828, 3293923677.75, 3293923688.062, 3293923722.5309997, 3293923726.64, 3293923730.671, 3293923734.843, 3293923739.015, 3293923743.437, 3293923747.437], [0.02463431842625141, 0.02463431842625141, 0.33257317543029785, -0.26877567172050476, -0.21053607761859894, -0.3878229558467865, -0.627870500087738, -0.627870500087738, -0.35187196731567383, 0.61182701587677, 0.414733350276947, 0.06820612400770187, 0.033184804022312164, 0.28442147374153137, 0.3806324601173401, 0.3806324601173401, -0.5958633422851562, -0.5958633422851562, -0.3973797857761383, 0.1421676129102707, 0.1421676129102707, 0.390238881111145, 0.4161102771759033, 0.6681324243545532, 0.08439777046442032, 0.12898856401443481, 0.07825367152690887, -0.09022828936576843, -0.0057562836445868015, -0.2819269895553589, -0.21260638535022736, 0.050426241010427475, -0.3064248561859131, 0.3770900368690491, 0.3633768482208252]}] caption="Graphique du Flux de l'étoile guide"
  out "Connexion LVDTs":bool
  out "Connexion Météo":bool
  out "PrAMS + Hexapode":bool
  out "Astrométries":bool
  out "Vitesse des tables":bool
  out "Choix de l'insturment":bool
  out "Initialisation TCS":bool
  out "Gestion des menus":bool
  out "Lecture Configuration":bool
  out "Vérification des erreurs":bool
  out "Événements Usagés":bool
  out "Stops":bool
  out "Synchro StarryNight":bool
  out "Query et Status":bool
  out "Événements Software":bool
  out "Guidage":bool
  out "Archivage SAOMM":bool
  out "PrAMS + SAOMM":bool
  out "PrAMS Listener":bool
  out "Hexapod Listener":bool
  out "Afficahge d'erreur":bool
  out "Scripts Listener":bool
  out "Gestion Scripts":bool
  in  "Quit":bool=TRUE caption="Sauvegarder et Quitter"
  out "Target OutofRange":bool
  out "Approaching limit":bool
  out "ModeInv":bool
  out "lampOn?":bool
  out "StarFaded?":bool
  out "FlatOn":bool caption="Flat"
  out "NeonOn":bool caption="Neon"
  out "ArcOn":bool caption="Arc"
  in  "Centre":bool
  out "ImageUsage":u16(ring) items=["Region d'intérêt", "Prévisualisation", "Idle"]
  out "Position Y":dbl=688453.0
  out "Position X":dbl=640645.0
  out "HexV":dbl caption="Position Hexapode 'V'" format="%.4f"
  out "HexU":dbl caption="Position Hexapode 'V'" format="%.4f"
  out "HexZ":dbl caption="Position Hexapode 'Z'" format="%.4f"
  out "HexY":dbl caption="Position Hexapode 'Y'" format="%.4f"
  out "RotationTCS":dbl=90.0 caption="Angle du rotateur d'instrument" min=-120.0 max=120.0 step=1.0 format="%.1f"
  out "Saturé":bool
  out "HexX":dbl caption="Position HExapode 'X'" format="%.4f"
  in  "Rechercher...":string
  out "Librairie des objets":string[][](table)=[["1", "WR1", "00:43:28", "64:45:35", "2000.0", "1.153488"], ["2", "WR2", "01:05:23", "60:25:18", "2000.0", "1.142985"], ["3", "WR3", "02:54:30", "-10:00:17", "2006.2", "2.742240"], ["4", "WR4", "02:00:00", "10:00:00", "2000.0", "1.613543"], ["5", "WR5", "02:52:11", "56:56:07", "2000.0", "1.148727"], ["6", "WR6", "06:54:13", "-23:55:42", "2000.0", "7.346970"], ["7", "WR7", "07:18:29", "-13:13:01", "2000.0", "3.540250"], ["8", "WR7a", "07:20:22", "-23:43:57", "2000.0", "7.387993"], ["9", "WR8", "07:44:58", "-31:54:29", "2000.0", "29.253050"]]
  out "TERMINAL":string="### ### ### ### ### ### ### ### ###\n\n     Démarrage du programme !  Bonne nuit !\n\n### ### ### ### ### ### ### ### ###\r2008-09-24, 00:01 #: Lancement de \"Errorcheck.vi\"\r2008-09-24, 00:02 #: Initialisation des variables\r2008-09-24, 00:02 #: Test des commandes TCS\r2008-09-24, 00:02 #: Changement du périphérique pour \"Options des périphériques\"\r2008-09-24, 00:02 #: Changement du mode de la caméra pour \"Exposition simple\"\r2008-09-24, 00:02 #: Changement du périphérique pour \"Roue à Filtres (BonOMM)\"\r2008-09-24, 00:02 #: Modification de la liste des filtres\r2008-09-24, 00:03 #: Arrêt du guidage\r2008-09-24, 00:03 #: Arrêt de la caméra de guidage, état : connectée"
  in  "Load-library":bool caption="Charger une librarie"
  in  "load-histo(L)":bool caption="Charger l'objet sélectionné"
  in  "Classé par ...":i32(ring) items=["Index", "Pseudo", "RA", "DEC", "Epoch", "Airmass"]
  out "Indicateur d'état":string="Lecture des paramètres des tables"
  out "HexTemp COMM":bool=TRUE
  in  "HexTemp VRN":refnum<visa-resource-name>="COM8"
  in  "HexTemp Baud rate":u32=38400
  out "TrackLogFilename":string
  out "Splitter COMM":bool=TRUE
  in  "Splitter VRN":refnum<visa-resource-name>="COM8"
  in  "Splitter Baud rate":u32=38400
  out "Hexapod COMM":bool=TRUE
  out "CmdDone":T14(array[cluster]) caption="Commandes Effectuées"
  in  "Port Local":u16
  in  "MCB Baud Rate":u32=57600
  out "Warning Code":u32
  in  "ANSW":string
  out "ActiveCmd":T15 caption="Commande Active"
  in  "TCS VRN":refnum<visa-resource-name>="COM7" caption="ID de connexion WinTCS"
  in  "PrAMS VRN":refnum<visa-resource-name>="COM4" caption="ID de connexion PrAMS"
  in  "MC-BonOMM VRN":refnum<visa-resource-name>="COM3"
  out "MCB COMM":bool=TRUE
  out "TCS COMM":bool=TRUE
  out "CmdPending":bool caption="Commande Active ?"
  out "CmdFIFO":T14(array[cluster]) caption="Commandes Latentes"
  out "Error Code":u32
  out "path_exclusion":path=path "C:/BonOMM/BonOMM 7.1/systemlogfiles" caption="Chemin du fichier d'exclusion"
  out "VI principal":path=path "C:/BonOMM/BonOMM 7.1/BonOMM 7.1.vi" caption="Chemin du dossier principal"
  out "path_config":path=path "C:/BonOMM/BonOMM 7.1/BonOMM 7.1.vi" caption="Répertoire de configuration"
  out "properties.ini":path=path "C:/BonOMM/BonOMM 7.1/BonOMM 7.1.vi" caption="Fichier de Configuration Système"
